vi "Frisbee Vision Processing.vi"(1 "Number of Particles (Particle Analysis 1)":i32, 4 "Particle Measurements (Pixels) (Particle Analysis 1)":dbl[][](array[numeric]) format="%.2f", 11 "Circles Data (Circle Detection 1)":T3(array[cluster])) -> (10 "Chosen Particle Info":T2, 12 "Ordered Pairs":T1, 13 "Number of Pairs":i32, 14 "Intercept":dbl, 19 "Slope Angle":dbl)   [LabVIEW 2012]
uses:
  <vilib>/Analysis/Matrix/Datatypes/RealMatrix.ctl
  <vilib>/Analysis/Matrix/Numeric/Conversions/Array To Matrix - RA2.vi
  <vilib>/Analysis/Matrix/NI_Matrix.lvlib
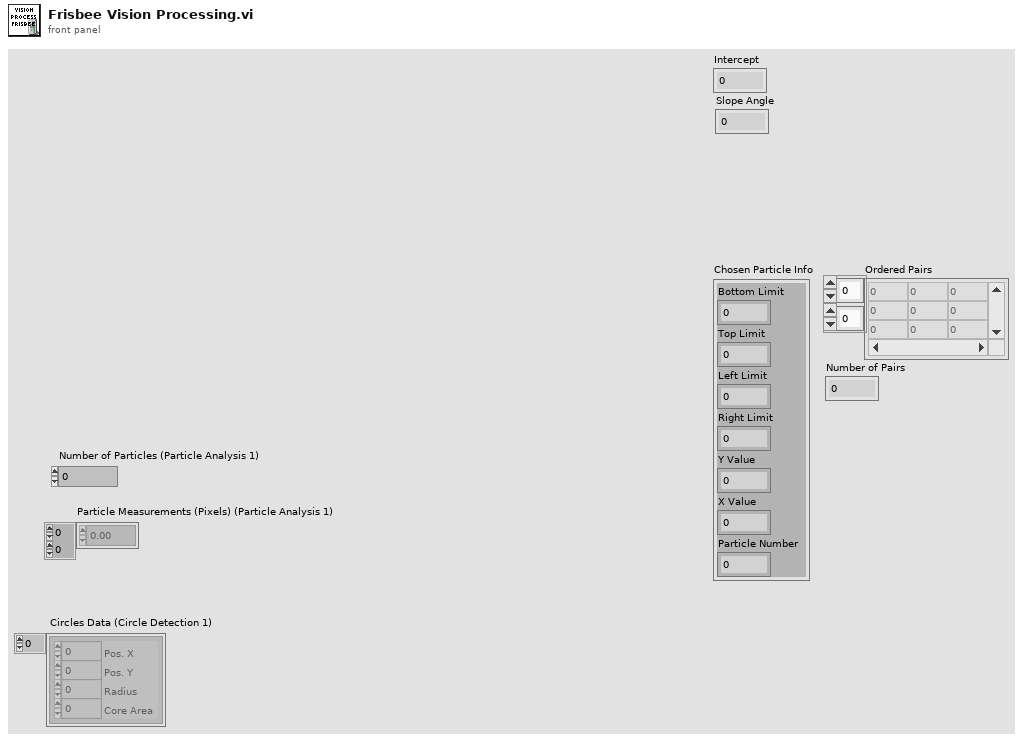
[diagram p1: front panel]
types:
  T1 = typedef "NI_Matrix.lvlib/RealMatrix.ctl" = dbl[][]
  T2 = cluster{"Bottom Limit":i32, "Top Limit":i32, "Left Limit":i32, "Right Limit":i32, "Y Value":i32, "X Value":i32, "Particle Number":i32}
  T3 = cluster{"Pos. X":i32, "Pos. Y":i32, "Radius":i32, "Core Area":i32}[]
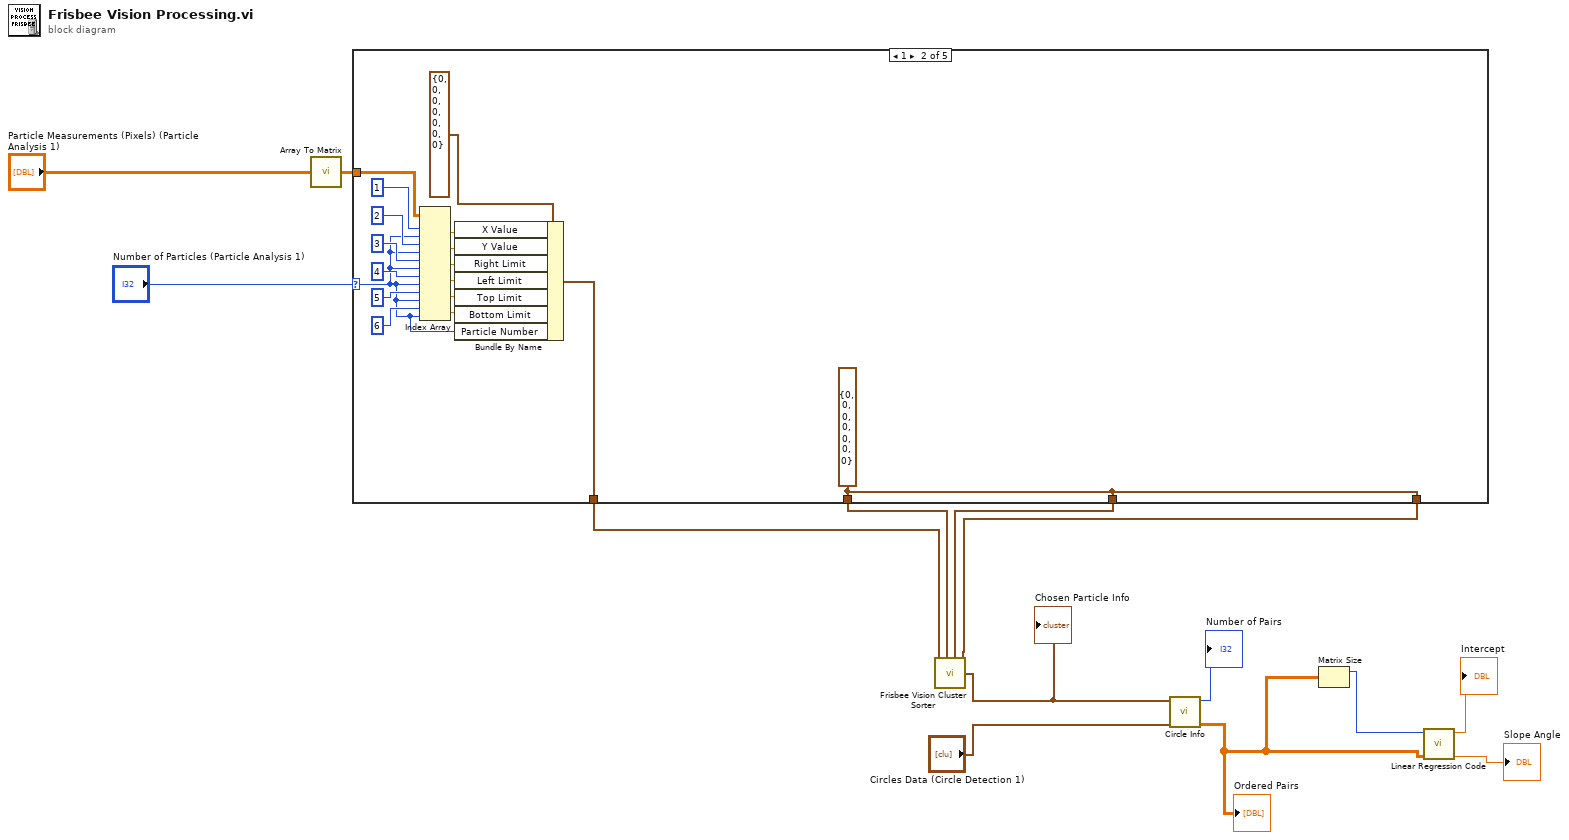
[diagram p0: block diagram]
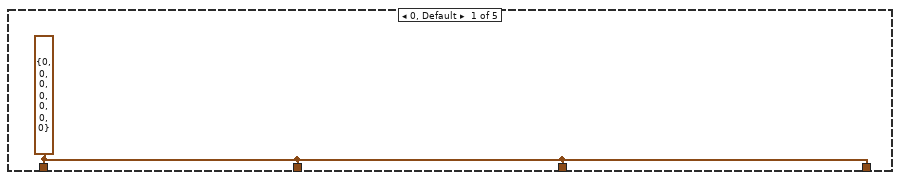
[diagram p2: hidden frame]
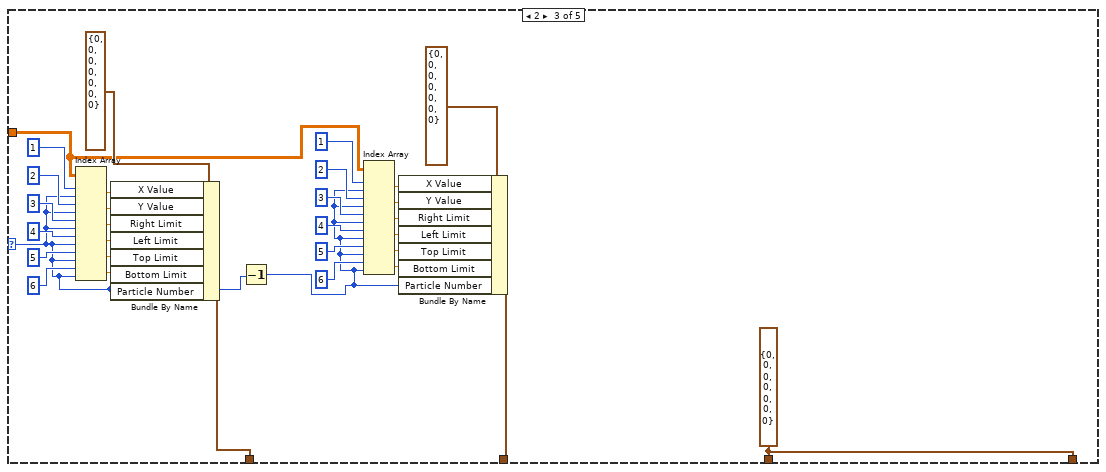
[diagram p3: hidden frame]
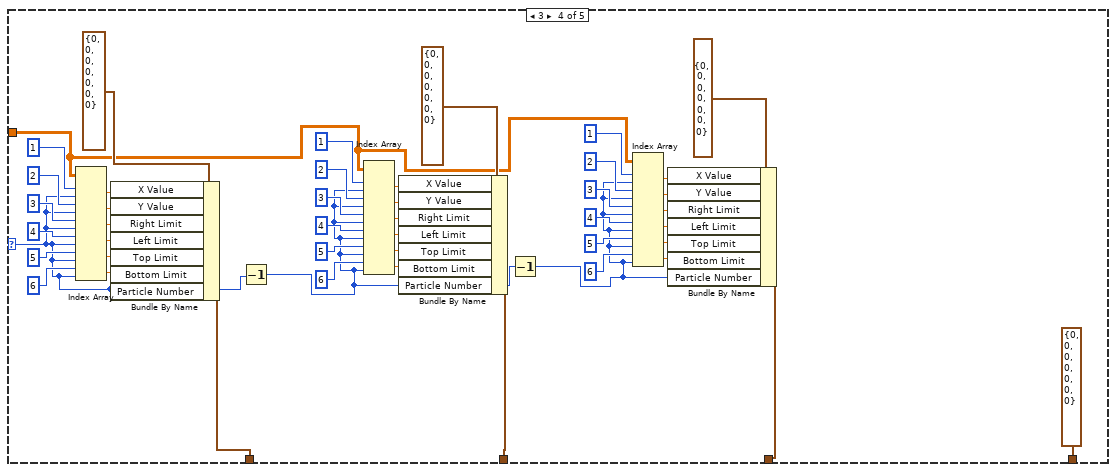
[diagram p4: hidden frame]
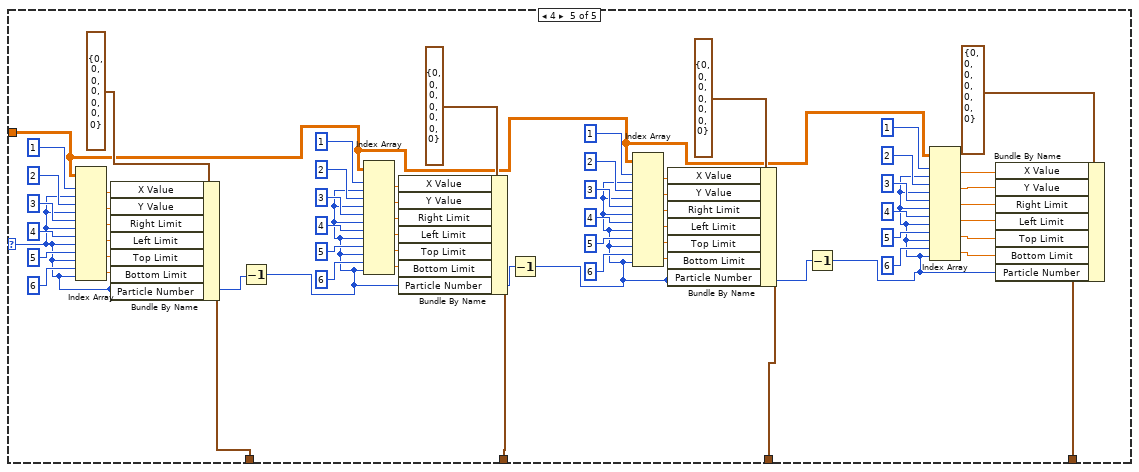
[diagram p5: hidden frame]
diagram:
  n1 = call-poly <vilib>:"Array To Matrix.vi"("Real 2D Array"="Particle Measurements (Pixels) (Particle Analysis 1)") -> ("Real Matrix"=w12:T1)
  n2 = case shown="1" "Number of Particles (Particle Analysis 1)" {
    selector: "Number of Particles (Particle Analysis 1)" -> [_ w16 w34 w67 w116]
    tunnel: w12 -> [_ w32 w40 w72 w121]
    tunnel: [w15 w18 w37 w71 w120] -> w11
    tunnel: [w15 w17 w36 w70 w119] -> w10
    tunnel: [w15 w17 w35 w69 w118] -> w9
    tunnel: [w15 w17 w35 T2 {"Bottom Limit"=0, "Top Limit"=0, "Left Limit"=0, "Right Limit"=0, "Y Value"=0, "X Value"=0, "Particle Number"=0} ("input cluster") w117] -> w8
    frame 0, Default {
      w15 = T2 {"Bottom Limit"=0, "Top Limit"=0, "Left Limit"=0, "Right Limit"=0, "Y Value"=0, "X Value"=0, "Particle Number"=0} ("input cluster")
    }
    frame 1 {
      w17 = T2 {"Bottom Limit"=0, "Top Limit"=0, "Left Limit"=0, "Right Limit"=0, "Y Value"=0, "X Value"=0, "Particle Number"=0} ("input cluster")
      n3 = Index Array(array=w32, index (row) #1=1 ("index (row)"), index (col) #1=w16, index (row) #2=2 ("index (row)"), index (col) #2=w16, index (row) #3=3 ("index (row)"), index (col) #3=w16, index (row) #4=4 ("index (row)"), index (col) #4=w16, index (row) #5=5 ("index (row)"), index (col) #5=w16, index (row) #6=6 ("index (row)"), index (col) #6=w16) -> (element #1=w20:dbl, element #2=w25:dbl, element #3=w24:dbl, element #4=w23:dbl, element #5=w22:dbl, element #6=w19:dbl)
      n4 = Bundle By Name(cluster=T2 {"Bottom Limit"=0, "Top Limit"=0, "Left Limit"=0, "Right Limit"=0, "Y Value"=0, "X Value"=0, "Particle Number"=0} ("input cluster"), "X Value"=w20, "Y Value"=w25, "Right Limit"=w24, "Left Limit"=w23, "Top Limit"=w22, "Bottom Limit"=w19, "Particle Number"=w16) -> (w18:T2)
    }
    frame 2 {
      w35 = T2 {"Bottom Limit"=0, "Top Limit"=0, "Left Limit"=0, "Right Limit"=0, "Y Value"=0, "X Value"=0, "Particle Number"=0} ("input cluster")
      n5 = Index Array(array=w40, index (row) #1=1 ("index (row)"), index (col) #1=w34, index (row) #2=2 ("index (row)"), index (col) #2=w34, index (row) #3=3 ("index (row)"), index (col) #3=w34, index (row) #4=4 ("index (row)"), index (col) #4=w34, index (row) #5=5 ("index (row)"), index (col) #5=w34, index (row) #6=6 ("index (row)"), index (col) #6=w34) -> (element #1=w53:dbl, element #2=w58:dbl, element #3=w57:dbl, element #4=w56:dbl, element #5=w55:dbl, element #6=w52:dbl)
      n6 = Bundle By Name(cluster=T2 {"Bottom Limit"=0, "Top Limit"=0, "Left Limit"=0, "Right Limit"=0, "Y Value"=0, "X Value"=0, "Particle Number"=0} ("input cluster"), "X Value"=w53, "Y Value"=w58, "Right Limit"=w57, "Left Limit"=w56, "Top Limit"=w55, "Bottom Limit"=w52, "Particle Number"=w34) -> (w37:T2)
      n7 = Decrement(x=w34) -> (x-1=w33:i32)
      n8 = Index Array(array=w40, index (row) #1=1 ("index (row)"), index (col) #1=w33, index (row) #2=2 ("index (row)"), index (col) #2=w33, index (row) #3=3 ("index (row)"), index (col) #3=w33, index (row) #4=4 ("index (row)"), index (col) #4=w33, index (row) #5=5 ("index (row)"), index (col) #5=w33, index (row) #6=6 ("index (row)"), index (col) #6=w33) -> (element #1=w42:dbl, element #2=w46:dbl, element #3=w45:dbl, element #4=w44:dbl, element #5=w43:dbl, element #6=w41:dbl)
      n9 = Bundle By Name(cluster=T2 {"Bottom Limit"=0, "Top Limit"=0, "Left Limit"=0, "Right Limit"=0, "Y Value"=0, "X Value"=0, "Particle Number"=0} ("input cluster"), "X Value"=w42, "Y Value"=w46, "Right Limit"=w45, "Left Limit"=w44, "Top Limit"=w43, "Bottom Limit"=w41, "Particle Number"=w33) -> (w36:T2)
    }
    frame 3 {
      n10 = Index Array(array=w72, index (row) #1=1 ("index (row)"), index (col) #1=w67, index (row) #2=2 ("index (row)"), index (col) #2=w67, index (row) #3=3 ("index (row)"), index (col) #3=w67, index (row) #4=4 ("index (row)"), index (col) #4=w67, index (row) #5=5 ("index (row)"), index (col) #5=w67, index (row) #6=6 ("index (row)"), index (col) #6=w67) -> (element #1=w100:dbl, element #2=w105:dbl, element #3=w104:dbl, element #4=w103:dbl, element #5=w102:dbl, element #6=w99:dbl)
      n11 = Bundle By Name(cluster=T2 {"Bottom Limit"=0, "Top Limit"=0, "Left Limit"=0, "Right Limit"=0, "Y Value"=0, "X Value"=0, "Particle Number"=0} ("input cluster"), "X Value"=w100, "Y Value"=w105, "Right Limit"=w104, "Left Limit"=w103, "Top Limit"=w102, "Bottom Limit"=w99, "Particle Number"=w67) -> (w71:T2)
      n12 = Decrement(x=w67) -> (x-1=w66:i32)
      n13 = Index Array(array=w72, index (row) #1=1 ("index (row)"), index (col) #1=w66, index (row) #2=2 ("index (row)"), index (col) #2=w66, index (row) #3=3 ("index (row)"), index (col) #3=w66, index (row) #4=4 ("index (row)"), index (col) #4=w66, index (row) #5=5 ("index (row)"), index (col) #5=w66, index (row) #6=6 ("index (row)"), index (col) #6=w66) -> (element #1=w89:dbl, element #2=w93:dbl, element #3=w92:dbl, element #4=w91:dbl, element #5=w90:dbl, element #6=w88:dbl)
      n14 = Bundle By Name(cluster=T2 {"Bottom Limit"=0, "Top Limit"=0, "Left Limit"=0, "Right Limit"=0, "Y Value"=0, "X Value"=0, "Particle Number"=0} ("input cluster"), "X Value"=w89, "Y Value"=w93, "Right Limit"=w92, "Left Limit"=w91, "Top Limit"=w90, "Bottom Limit"=w88, "Particle Number"=w66) -> (w70:T2)
      n15 = Decrement(x=w66) -> (x-1=w65:i32)
      n16 = Index Array(array=w72, index (row) #1=1 ("index (row)"), index (col) #1=w65, index (row) #2=2 ("index (row)"), index (col) #2=w65, index (row) #3=3 ("index (row)"), index (col) #3=w65, index (row) #4=4 ("index (row)"), index (col) #4=w65, index (row) #5=5 ("index (row)"), index (col) #5=w65, index (row) #6=6 ("index (row)"), index (col) #6=w65) -> (element #1=w76:dbl, element #2=w80:dbl, element #3=w79:dbl, element #4=w78:dbl, element #5=w77:dbl, element #6=w75:dbl)
      n17 = Bundle By Name(cluster=T2 {"Bottom Limit"=0, "Top Limit"=0, "Left Limit"=0, "Right Limit"=0, "Y Value"=0, "X Value"=0, "Particle Number"=0} ("input cluster"), "X Value"=w76, "Y Value"=w80, "Right Limit"=w79, "Left Limit"=w78, "Top Limit"=w77, "Bottom Limit"=w75, "Particle Number"=w65) -> (w69:T2)
    }
    frame 4 {
      n18 = Index Array(array=w121, index (row) #1=1 ("index (row)"), index (col) #1=w116, index (row) #2=2 ("index (row)"), index (col) #2=w116, index (row) #3=3 ("index (row)"), index (col) #3=w116, index (row) #4=4 ("index (row)"), index (col) #4=w116, index (row) #5=5 ("index (row)"), index (col) #5=w116, index (row) #6=6 ("index (row)"), index (col) #6=w116) -> (element #1=w161:dbl, element #2=w166:dbl, element #3=w165:dbl, element #4=w164:dbl, element #5=w163:dbl, element #6=w160:dbl)
      n19 = Bundle By Name(cluster=T2 {"Bottom Limit"=0, "Top Limit"=0, "Left Limit"=0, "Right Limit"=0, "Y Value"=0, "X Value"=0, "Particle Number"=0} ("input cluster"), "X Value"=w161, "Y Value"=w166, "Right Limit"=w165, "Left Limit"=w164, "Top Limit"=w163, "Bottom Limit"=w160, "Particle Number"=w116) -> (w120:T2)
      n20 = Decrement(x=w116) -> (x-1=w115:i32)
      n21 = Index Array(array=w121, index (row) #1=1 ("index (row)"), index (col) #1=w115, index (row) #2=2 ("index (row)"), index (col) #2=w115, index (row) #3=3 ("index (row)"), index (col) #3=w115, index (row) #4=4 ("index (row)"), index (col) #4=w115, index (row) #5=5 ("index (row)"), index (col) #5=w115, index (row) #6=6 ("index (row)"), index (col) #6=w115) -> (element #1=w150:dbl, element #2=w154:dbl, element #3=w153:dbl, element #4=w152:dbl, element #5=w151:dbl, element #6=w149:dbl)
      n22 = Bundle By Name(cluster=T2 {"Bottom Limit"=0, "Top Limit"=0, "Left Limit"=0, "Right Limit"=0, "Y Value"=0, "X Value"=0, "Particle Number"=0} ("input cluster"), "X Value"=w150, "Y Value"=w154, "Right Limit"=w153, "Left Limit"=w152, "Top Limit"=w151, "Bottom Limit"=w149, "Particle Number"=w115) -> (w119:T2)
      n23 = Decrement(x=w115) -> (x-1=w114:i32)
      n24 = Index Array(array=w121, index (row) #1=1 ("index (row)"), index (col) #1=w114, index (row) #2=2 ("index (row)"), index (col) #2=w114, index (row) #3=3 ("index (row)"), index (col) #3=w114, index (row) #4=4 ("index (row)"), index (col) #4=w114, index (row) #5=5 ("index (row)"), index (col) #5=w114, index (row) #6=6 ("index (row)"), index (col) #6=w114) -> (element #1=w137:dbl, element #2=w141:dbl, element #3=w140:dbl, element #4=w139:dbl, element #5=w138:dbl, element #6=w136:dbl)
      n25 = Bundle By Name(cluster=T2 {"Bottom Limit"=0, "Top Limit"=0, "Left Limit"=0, "Right Limit"=0, "Y Value"=0, "X Value"=0, "Particle Number"=0} ("input cluster"), "X Value"=w137, "Y Value"=w141, "Right Limit"=w140, "Left Limit"=w139, "Top Limit"=w138, "Bottom Limit"=w136, "Particle Number"=w114) -> (w118:T2)
      n26 = Decrement(x=w114) -> (x-1=w113:i32)
      n27 = Index Array(array=w121, index (row) #1=1 ("index (row)"), index (col) #1=w113, index (row) #2=2 ("index (row)"), index (col) #2=w113, index (row) #3=3 ("index (row)"), index (col) #3=w113, index (row) #4=4 ("index (row)"), index (col) #4=w113, index (row) #5=5 ("index (row)"), index (col) #5=w113, index (row) #6=6 ("index (row)"), index (col) #6=w113) -> (element #1=w112:dbl, element #2=w128:dbl, element #3=w127:dbl, element #4=w126:dbl, element #5=w125:dbl, element #6=w124:dbl)
      n28 = Bundle By Name(cluster=T2 {"Bottom Limit"=0, "Top Limit"=0, "Left Limit"=0, "Right Limit"=0, "Y Value"=0, "X Value"=0, "Particle Number"=0} ("input cluster"), "X Value"=w112, "Y Value"=w128, "Right Limit"=w127, "Left Limit"=w126, "Top Limit"=w125, "Bottom Limit"=w124, "Particle Number"=w113) -> (w117:T2)
    }
  }
  n29 = call "Frisbee Vision Cluster Sorter.vi"("input cluster"=w11, "input cluster 2"=w10, "input cluster 3"=w9, "input cluster 4"=w8) -> ("Chosen Particle Info"=w7:T2)  [unwired: 5 in]
  "Chosen Particle Info" <- w7
  n30 = call "Circle Info.vi"("Circles Data (Circle Detection 1) 2"="Circles Data (Circle Detection 1)", "Chosen Particle Info 2"=w7) -> ("Ordered Pairs"=w4:T1, "Number of Pairs"=→"Number of Pairs":i32)  [unwired: 8 in]
  "Ordered Pairs" <- w4
  n31 = Matrix Size(0:w4) -> (1:w3:i32)  [unwired: 1 out]
  n32 = call "Linear Regression Code.vi"("Ordered Pairs"=w4, "Number of Pairs"=w3) -> ("Slope Angle"=→"Slope Angle":dbl, "Intercept"=→"Intercept":dbl)  [unwired: 7 in]
